vi "Fluke 884X Series Read Triggered Multiple.vi"() -> ()   [LabVIEW 2010]
doc: "This example shows how to configure a measurement, set up triggering, trigger a measurement, and retrieve a measurement. It shows how to use the low-level Data VIs to retrieve data from the DMM.\n\n<B>Note:</B>\n\nThe product of the Sample Count and Trigger Count must not exceed 5000 readings since it uses low level VIs (<B>Initiate</B> and <B>Fetch</B>) that have a 5000 point internal memory limitation."
uses:
  <vilib>/Utility/error.llb/DialogType.ctl
  <instrlib>/Fluke 884X Series/Fluke 884X Series.lvlib
panel:
  in  "Timeout (10000 ms)":u32=10000
  in  "Sample Count (10)":i32=10 format="%#.6g"
  out "Waveform Chart":dbl[](graph)
  in  "Trigger Count (5)":i32=5 format="%#.6g"
  in  "Function (0: DC Voltage)":u16(ring) items=["DC Voltage", "AC Voltage", "2 - Wire Resistance", "4 - Wire Resistance", "DC Current", "AC Current", "Frequency", "Period", "Continuity", "Diode Checking", "Temperature", "Capacitance"]
  in  "Serial Configuration":T1={"Baud Rate"=9600, "Parity"=0, "Data Bits"=8, "Stop Bits"=10, "Flow Control"=0} {"Flow Control" items=["None", "XON/XOFF", "RTS/CTS", "XON/XOFF & RTS/CTS", "DTR/DSR", "XON/XOFF & DTR/DSR"]; "Stop Bits" items=["1.0"=10, "1.5"=15, "2.0"=20]; "Data Bits" items=["7"=7, "8"=8]; "Parity" items=["None", "Odd", "Even", "Mark", "Space"]; "Baud Rate" items=["300"=300, "600"=600, "1200"=1200, "2400"=2400, "4800"=4800, "9600"=9600, "19200"=19200]}
  in  "VISA resource name":refnum<visa-resource-name>
  # "(c) 2007 National Instruments.  ALL RIGHTS RESERVED."
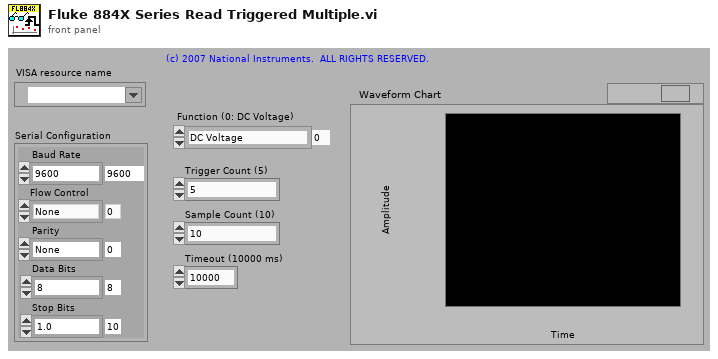
[diagram p1: front panel]
types:
  T1 = cluster{"Baud Rate":u32, "Parity":u16, "Data Bits":u16, "Stop Bits":u16, "Flow Control":u16}
  T2 = typedef "DialogType.ctl" = u16
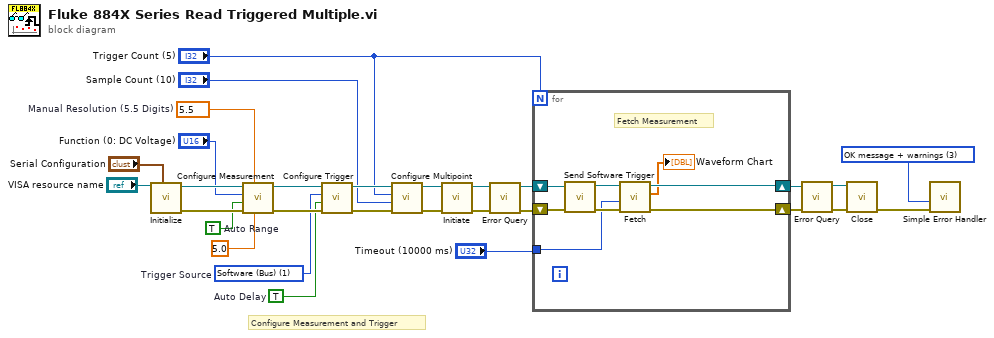
[diagram p0: block diagram]
diagram:
  w3 = 5.5 items=["4.5"=4.5, "5.5"=5.5, "6.5"=6.5]  # Manual Resolution (5.5 Digits)
  w11 = TRUE  # Auto Delay
  w12 = u16 1 items=["Immediate", "Software (Bus)", "External"]  # Trigger Source
  w13 = TRUE  # Auto Range
  w16 = T2 3 items=["no dialog", "OK message", "continue or stop message", "OK message + warnings", "continue/stop + warnings"] ("type of dialog (OK msg:1)")
  # "Configure Measurement and Trigger"
  n1 = call <instrlib>:"Initialize.vi"("Serial Configuration"="Serial Configuration", "VISA resource name"="VISA resource name") -> ("error out"=w28:errorcluster, "VISA resource name out"=w29:refnum<visa-resource-name>)  [unwired: 8 in]
  n2 = call <instrlib>:"Configure Measurement.vi"("Manual Range (1.0)"=5.0, "Manual Resolution (5.5 Digits)"=w3, "error in (no error)"=w28, "Auto Range (T:Enable)"=w13, "Function (0: DC Voltage)"="Function (0: DC Voltage)", "VISA resource name"=w29) -> ("error out"=w26:errorcluster, "VISA resource name out"=w27:refnum<visa-resource-name>)  [unwired: 4 in]
  n3 = call <instrlib>:"Configure Trigger.vi"("error in (no error)"=w26, "Auto Delay (T: Enable)"=w11, "Trigger Source (0: Immediate)"=w12, "VISA resource name"=w27) -> ("error out"=w24:errorcluster, "VISA resource name out"=w25:refnum<visa-resource-name>)  [unwired: 6 in]
  n4 = call <instrlib>:"Configure Multipoint.vi"("error in (no error)"=w24, "Sample Count (1)"="Sample Count (10)", "Trigger Count (1)"="Trigger Count (5)", "VISA resource name"=w25) -> ("error out"=w21:errorcluster, "VISA resource name out"=w22:refnum<visa-resource-name>)  [unwired: 6 in]
  n5 = call <instrlib>:"Initiate.vi"("error in (no error)"=w21, "VISA resource name"=w22) -> ("error out"=w8:errorcluster, "VISA resource name out"=w7:refnum<visa-resource-name>)  [unwired: 8 in]
  n6 = call <instrlib>:"Error Query.vi"("error in (no error)"=w8, "VISA resource name"=w7) -> ("error out"=w5:errorcluster, "VISA resource name out"=w6:refnum<visa-resource-name>)  [unwired: 6 in, 2 out]
  n7 = for {
    N: "Trigger Count (5)" -> [_]
    shift-right: [w36] -> w18
    shift-left: w5 -> [w32]
    shift-right: [w37] -> w20
    shift-left: w6 -> [w33]
    tunnel: "Timeout (10000 ms)" -> [w31]
    # "Fetch Measurement"
    n8 = call <instrlib>:"Send Software Trigger.vi"("error in (no error)"=w32, "VISA resource name"=w33) -> ("error out"=w34:errorcluster, "VISA resource name out"=w35:refnum<visa-resource-name>)  [unwired: 8 in]
    n9 = call <instrlib>:"Fetch.vi"("error in (no error)"=w34, "Timeout (10000 ms)"=w31, "VISA resource name"=w35) -> ("error out"=w36:errorcluster, "Measurements"=→"Waveform Chart":dbl[], "VISA resource name out"=w37:refnum<visa-resource-name>)  [unwired: 6 in]
  }
  n10 = call <instrlib>:"Error Query.vi"("error in (no error)"=w18, "VISA resource name"=w20) -> ("error out"=w17:errorcluster, "VISA resource name out"=w19:refnum<visa-resource-name>)  [unwired: 6 in, 2 out]
  n11 = call <instrlib>:"Close.vi"("error in (no error)"=w17, "VISA resource name"=w19) -> ("error out"=w23:errorcluster)  [unwired: 9 in]
  n12 = call <vilib>:"Simple Error Handler.vi"("type of dialog (OK msg:1)"=w16, "error in (no error)"=w23) -> ()  [unwired: 3 in, 5 out]
